vi "Dipper Fridge Resistance Measurement 1.9.vi"() -> ()   [LabVIEW 2011]
panel:
  out "read buffer":string
  out "appended array 3":dbl[](array[numeric])
  out "appended array 2":dbl[](array[numeric])
  in  "Time delay":dbl
  out "appended array":dbl[](array[numeric])
  out "Temperature Vs Time":cluster{dbl[], dbl[]}(graph)
  out "3He Pot":string
  in  "Sample Cell \nThermometer":bool
  out "Current Resistance":string
  in  "error in (no error) 3":errorcluster
  out "Sample Cell":string
  in  "error in (no error)":errorcluster
  in  "Heater option":string
  in  "Lakeshore":bool
  out "Sample Vs. Temp":cluster{dbl[], dbl[]}(graph)
  out "Warning":string="Can't be smaller than 1 s"
  in  "Timer":bool caption="Reset"
  out "Time Elapsed":string
  in  "Save":bool
  out "var":i32
  in  "error in (no error) 2":errorcluster
  out "Heater":bool
  in  "Heater":bool
  out "Boolean":bool
  in  "Power":bool
  in  "Date format (0)":enum16{"short", "long", "abbreviated"}(ring)
  out "size (in bytes)":i64
  out "Calibration":cluster{dbl[], dbl[]}(graph)
  in  "File Path":path
  out "current time":timestamp
  out "Number of Data points":i32
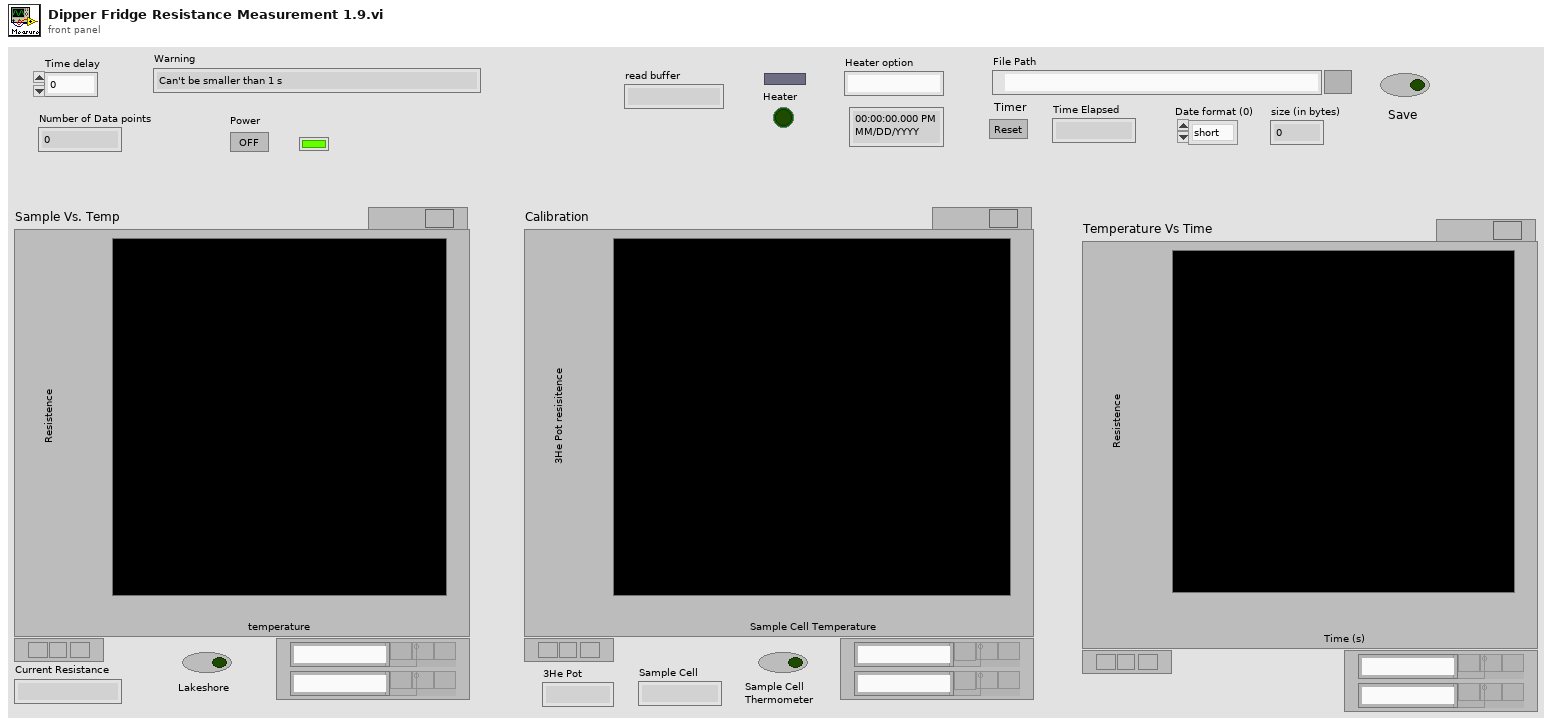
[diagram p1: front panel]
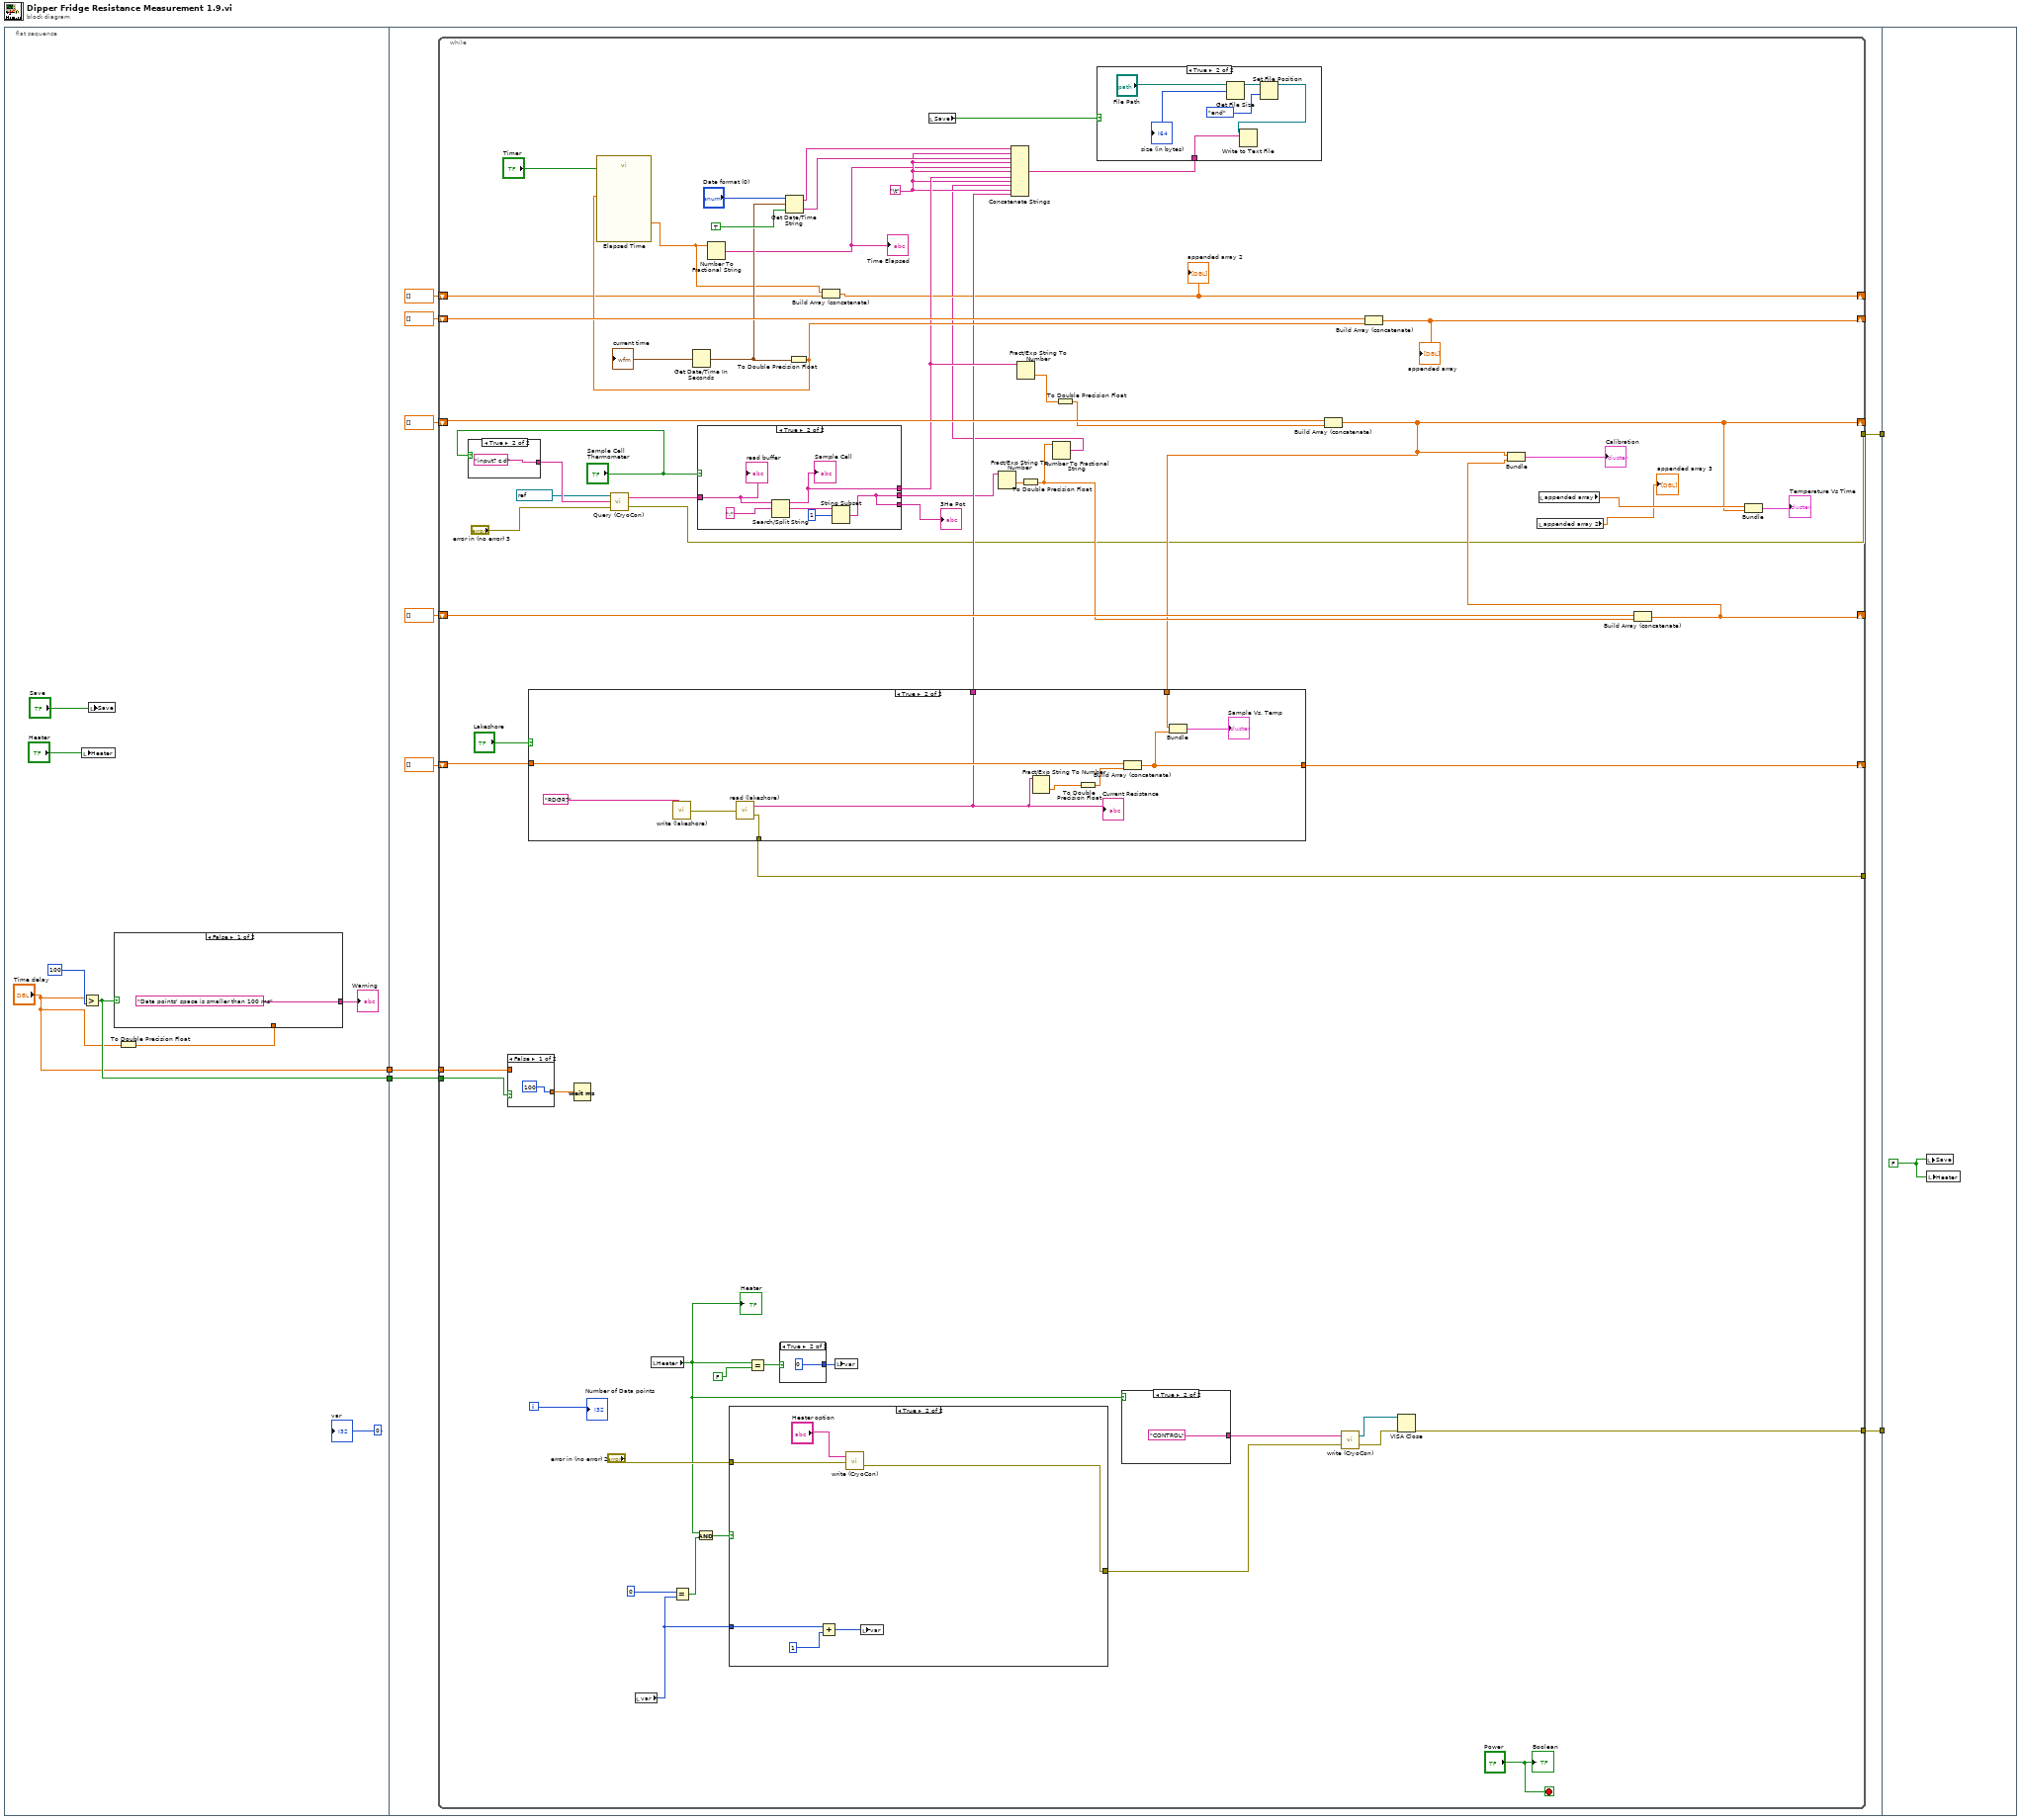
[diagram p0: block diagram]
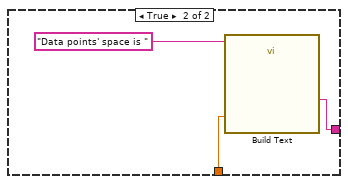
[diagram p2: hidden frame]
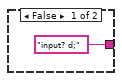
[diagram p3: hidden frame]
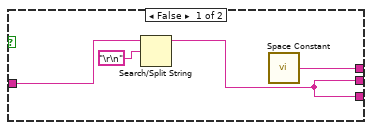
[diagram p4: hidden frame]
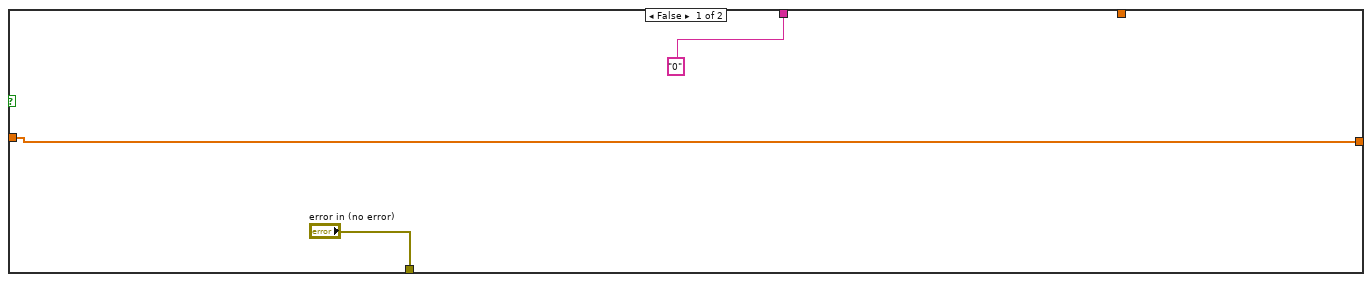
[diagram p5: hidden frame]
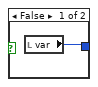
[diagram p7: hidden frame]
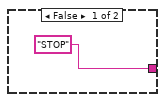
[diagram p9: hidden frame]
diagram:
  n1 = flat-sequence {
    tunnel: ["Time delay"] -> w4
    tunnel: [w6] -> w3
    tunnel: w4 -> [w21]
    tunnel: w3 -> [w20]
    tunnel: [w19] -> w2
    tunnel: [w18] -> w1
    tunnel: w2 -> [_]
    tunnel: w1 -> [_]
    frame #0 {
      n2 = local write "Heater"("Heater") -> ()
      n3 = Greater?(x="Time delay", y=u32 100 ("x")) -> (0:w6:bool)
      n4 = local write "Save"("Save") -> ()
      n5 = To Double Precision Float(number="Time delay") -> (double precision float=w7:dbl)
      n6 = case shown="False" w6 {
        tunnel: w7 -> [_ w14]
        tunnel: ["Data points' space is smaller than 100 ms" w16] -> w8
        frame False {
        }
        frame True {
          n7 = call "Build Text"("Beginning Text"="Data points' space is ", "Y"=w14) -> ("Result"=w16:string)  [unwired: 12 in, 1 out]
        }
      }
      "Warning" <- w8
      "var" <- 0 ("var")
    }
    frame #1 {
      n8 = while {
        tunnel: [w87] -> _
        shift-right: [w56] -> _
        shift-left: dbl[] [] -> [w84]
        shift-right: [w31] -> _
        shift-left: dbl[] [] -> [w81]
        shift-right: [w55] -> _
        shift-left: dbl[] [] -> [w61]
        shift-right: [w32] -> _
        shift-left: dbl[] [] -> [w60]
        tunnel: w21 -> [w57]
        tunnel: w20 -> [w58]
        tunnel: [w27] -> w19
        tunnel: [w48] -> w18
        shift-right: [w39] -> _
        shift-left: dbl[] [] -> [w40]
        i -> [w86]
        stop <- "Power" stop-if-true
        w44 = "\t"
        n9 = case shown="True" "Sample Cell \nThermometer" {
          tunnel: ["input? d;" "input? c,d"] -> w30
          frame False {
          }
          frame True {
          }
        }
        n10 = case shown="False" w58 {
          tunnel: [100 w114] -> w59
          tunnel: w57 -> [_ w114]
          frame False {
          }
          frame True {
          }
        }
        n11 = Wait (ms)(milliseconds to wait=w59) -> ()  [unwired: 1 out]
        n12 = call "Query (CryoCon).vi"("error in (no error)"="error in (no error) 3", "write buffer"=w30, "VISA resource name 2"=refnum<visa-resource-name> "COM3") -> ("error out"=w27:errorcluster, "read buffer"=w28:string)
        n13 = local read "var"() -> (w76:i32)
        n14 = local read "Heater"() -> (w67:bool)
        "Heater" <- w67
        n15 = Equal?(x=0, y=w76) -> (x = y?=w74:bool)
        n16 = Get Date/Time In Seconds() -> (seconds since 1Jan1904=w66:timestamp)
        "current time" <- w66
        n17 = And(x=w67, y=w74) -> (x .and. y?=w73:bool)
        n18 = case shown="True" "Sample Cell \nThermometer" {
          tunnel: w28 -> [w92 w96]
          tunnel: [w90 w94] -> w35
          tunnel: [w93 w95] -> w46
          tunnel: [w90 w94] -> w45
          frame False {
            n19 = Search/Split String(string=w92, search string/char (-)="\r\n") -> (substring before match=w90:string)  [unwired: 1 in, 2 out]
            n20 = call <vilib>:"Space Constant.vi"() -> ("String"=w93:string)
          }
          frame True {
            n21 = Search/Split String(string=w96, search string/char (-)=";") -> (substring before match=w95:string, match + rest of string=w98:string)  [unwired: 1 in, 1 out]
            "Sample Cell" <- w95
            n22 = String Subset(string=w98, offset (0)=1) -> (substring=w94:string)  [unwired: 1 in]
            "read buffer" <- w96
          }
        }
        "3He Pot" <- w45
        n23 = case shown="True" w73 {
          tunnel: [w117 w118] -> w72
          tunnel: "error in (no error) 2" -> [w117 w120]
          tunnel: w76 -> [_ w123]
          frame False {
          }
          frame True {
            n24 = Add(x=w123, y=1) -> (x+y=w121:i32)
            n25 = call "write (CryoCon).vi"("error in (no error)"=w120, "write buffer"="Heater option") -> ("error out"=w118:errorcluster)  [unwired: 1 out]
            n26 = local write "var"(w121) -> ()
          }
        }
        n27 = Equal?(x=w67, y=FALSE ("Heater")) -> (x = y?=w69:bool)
        n28 = case shown="True" w69 {
          tunnel: [w115 0] -> w68
          frame False {
            n29 = local read "var"() -> (w115:i32)
          }
          frame True {
          }
        }
        n30 = Get Date/Time String(date format (0)="Date format (0)", seconds (now)=w66, want seconds? (F)=TRUE) -> (date string=w62:string, time string=w63:string)
        n31 = To Double Precision Float(number=w66) -> (double precision float=w65:dbl)
        n32 = call "Elapsed Time"("Reset"="Timer", "Set Start Time (s)"=w65) -> ("Elapsed Time (s)"=w41:dbl)  [unwired: 10 in, 7 out]
        n33 = Number To Fractional String(number=w41) -> (F-format string=w42:string)  [unwired: 3 in]
        "Time Elapsed" <- w42
        n34 = Build Array (concatenate)(w41, w40) -> (w39:dbl[])
        "appended array 2" <- w39
        n35 = local write "var"(w68) -> ()
        n36 = local read "Save"() -> (w71:bool)
        n37 = Fract/Exp String To Number(string=w35) -> (number=w51:dbl)  [unwired: 3 in, 1 out]
        n38 = Fract/Exp String To Number(string=w46) -> (number=w54:dbl)  [unwired: 3 in, 1 out]
        n39 = To Double Precision Float(number=w51) -> (double precision float=w34:dbl)
        n40 = Number To Fractional String(number=w34) -> (F-format string=w33:string)  [unwired: 3 in]
        n41 = To Double Precision Float(number=w54) -> (double precision float=w53:dbl)
        n42 = case shown="True" w67 {
          tunnel: ["STOP" ("write buffer") "CONTROL" ("write buffer")] -> w78
          frame False {
          }
          frame True {
          }
        }
        n43 = Build Array (concatenate)(w81, w53) -> (w31:dbl[])
        n44 = case shown="True" "Lakeshore" {
          tunnel: ["error in (no error)" w112] -> w87
          tunnel: w61 -> [w101 w109]
          tunnel: ["0" ("read buffer") w108] -> w43
          tunnel: [w101 w105] -> w55
          tunnel: w31 -> [_ w103]
          frame False {
          }
          frame True {
            n45 = call "write (lakeshore).vi"("write buffer"="RDGR?") -> ("error out"=w111:errorcluster)  [unwired: 1 in]
            n46 = call "read (lakeshore).vi"("error in (no error)"=w111) -> ("read buffer"=w108:string, "error out"=w112:errorcluster)
            "Current Resistance" <- w108
            n47 = Fract/Exp String To Number(string=w108) -> (number=w107:dbl)  [unwired: 3 in, 1 out]
            n48 = To Double Precision Float(number=w107) -> (double precision float=w106:dbl)
            n49 = Build Array (concatenate)(w109, w106) -> (w105:dbl[])
            n50 = Bundle(w103, w105) -> (→"Sample Vs. Temp":cluster{dbl[], dbl[]})  [unwired: 1 in]
          }
        }
        n51 = Concatenate Strings(w62, w44, w63, w44, w42, w44, w46, w44, w33, w44, w43) -> (w83:string)
        n52 = case shown="True" w71 {
          tunnel: w83 -> [_ w131]
          frame False {
          }
          frame True {
            n53 = Get File Size(file="File Path") -> (refnum out=w129:refnum<file>, size (in bytes)=→"size (in bytes)":i64)  [unwired: 1 in, 1 out]
            n54 = Set File Position(refnum=w129, from (0:start)=enum16{"start", "end", "current"}."end") -> (refnum out=w128:refnum<file>)  [unwired: 2 in, 1 out]
            n55 = Write to Text File(file (use dialog)=w128, text=w131) -> ()  [unwired: 2 in, 3 out]
          }
        }
        n56 = call "write (CryoCon).vi"("error in (no error)"=w72, "write buffer"=w78) -> ("error out"=w49:errorcluster, "VISA resource name out"=w50:refnum<visa-resource-name>)
        n57 = Build Array (concatenate)(w84, w65) -> (w56:dbl[])
        "appended array" <- w56
        n58 = VISA Close(VISA resource name=w50, error in (no error)=w49) -> (error out=w48:errorcluster)
        n59 = local read "appended array 2"() -> (→"appended array 3":dbl[])
        n60 = local read "appended array"() -> (w37:dbl[])
        n61 = Build Array (concatenate)(w60, w34) -> (w32:dbl[])
        n62 = Bundle(w31, w32) -> (→"Calibration":cluster{dbl[], dbl[]})  [unwired: 1 in]
        n63 = Bundle("appended array"=w37, w31) -> (→"Temperature Vs Time":cluster{"appended array":dbl[], dbl[]})  [unwired: 1 in]
        "Number of Data points" <- w86
        "Boolean" <- "Power"
      }
    }
    frame #2 {
      w132 = FALSE ("Save")
      n64 = local write "Save"(w132) -> ()
      n65 = local write "Heater"(w132) -> ()
    }
  }
